vi "Proceed.vi"(7 "component is ready (Y)":bool=TRUE, 8 "error in (no error)":errorcluster, 10 "ProceedMessage":refnum<class "ProceedMessage.lvclass">, 11 "ExampleClassDScaffold in":refnum<class "ExampleClassDScaffold.lvclass">) -> (0 "error out":errorcluster, 2 "all observers are ready?":bool, 3 "ExampleClassDScaffold out":refnum<class "ExampleClassDScaffold.lvclass">)   [LabVIEW 2012, in "ExampleClassDScaffold.lvclass"]
doc: "The Proceed method is used to check if your component is ready. Also it checks if the observers are ready. When the observers and the component are ready, it sends the proceed to its observee. If it's the highest observee, it distributes a stop command."
uses:
  ExampleClassDScaffold.lvclass
  <vilib>/Distrio/Murmex/ProceedMessage/ProceedMessage.lvclass
  <vilib>/Distrio/Murmex/Murmex/Murmex.lvclass
panel:
  # "This method is called when the PROCEED\ntrigger is sent. \n\nOverride this method when your component needs to\nrespond to this trigger. \n\nCall parent for proper implementation"
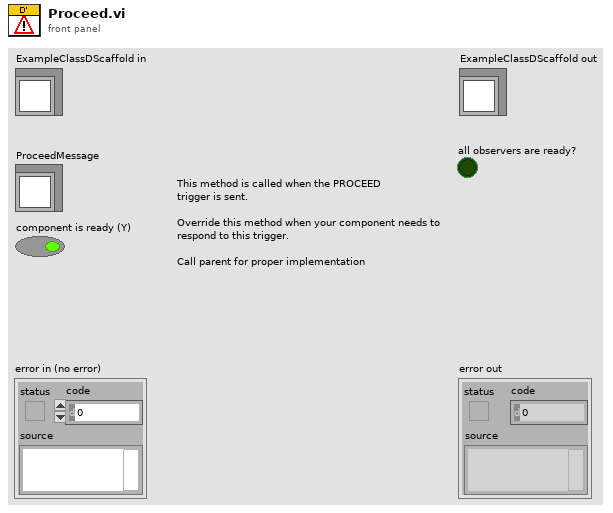
[diagram p1: front panel]
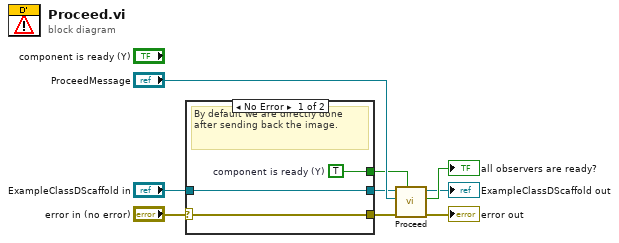
[diagram p0: block diagram]
diagram:
  n1 = case shown="No Error" "error in (no error)" {
    selector: "error in (no error)" -> [w10 w14]
    tunnel: [w12 _] -> w5
    tunnel: [w11 w13] -> w4
    tunnel: "ExampleClassDScaffold in" -> [w11 w13]
    tunnel: [w10 w14] -> w2
    frame No Error {
      w12 = TRUE  # component is ready (Y)
      # "By default we are directly done after sending back the image."
    }
    frame Error {
    }
  }
  n2 = call-parent "Proceed.vi"("component is ready (Y)"=w5, "error in (no error)"=w2, "ProceedMessage"="ProceedMessage", "Murmex in"=w4) -> ("error out"=→"error out":errorcluster, "all observers are ready?"=→"all observers are ready?":bool, "Murmex out"=→"ExampleClassDScaffold out":refnum<class "ExampleClassDScaffold.lvclass">)  [unwired: 5 in]
